vi "Create UI.vi"(8 "error in (no error)":errorcluster, 10 "Instrument.Example in":refnum<class "Instrument.lvclass">, 11 "Instrument.Example UI in":refnum<class "Instrument.PPMS2 UI.lvclass">) -> (0 "error out":errorcluster, 3 "Instrument.Example UI out":refnum<class "Instrument.PPMS2 UI.lvclass">)   [LabVIEW 2016, in "Instrument.PPMS2 UI.lvclass"]
uses:
  Instrument.PPMS2 UI.lvclass
  C:/Program Files (x86)/National Instruments/LabVIEW 2016/vi.lib/JKI/JKI SMO/SMO/SMO.lvclass
  <userlib>/LevyLab/Levylab Instruments/SMOs/Instrument/Instrument.lvclass
  Instrument.PPMS2 UI.lvclass/Instrument.PPMS2 UI.ctl
  <vilib>/JKI/JKI SMO/SMO/SMO.lvclass
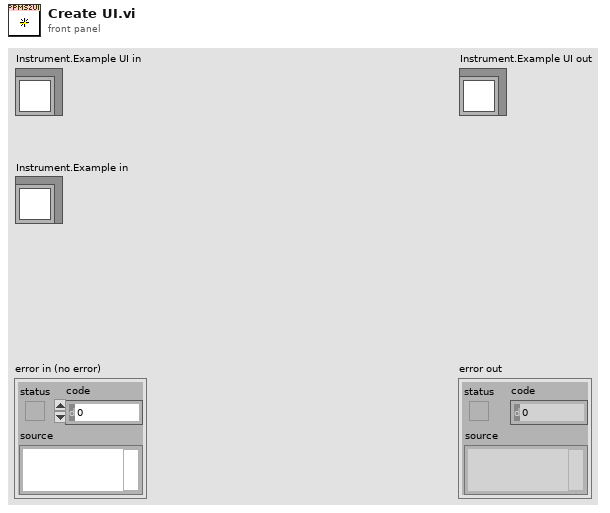
[diagram p1: front panel]
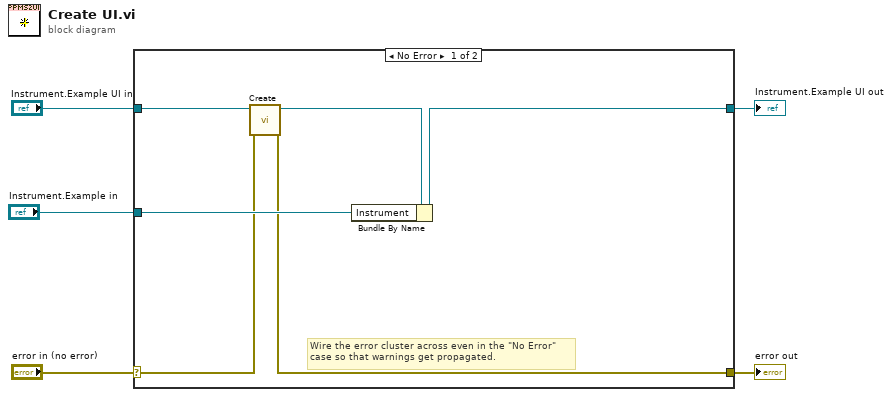
[diagram p0: block diagram]
diagram:
  n1 = case shown="No Error" "error in (no error)" {
    selector: "error in (no error)" -> [w7 w13]
    tunnel: [w6 w13] -> w4
    tunnel: [w11 w12] -> w2
    tunnel: "Instrument.Example UI in" -> [w9 w12]
    tunnel: "Instrument.Example in" -> [w10 _]
    frame No Error {
      # "Wire the error cluster across even in the \"No Error\"\ncase so that warnings get propagated."
      n2 = call <vilib>:"Create.vi"("error in (no error)"=w7, "SMO"=w9) -> ("error out"=w6:errorcluster, "SMO out"=w8:refnum<class "Instrument.PPMS2 UI.lvclass">)  [unwired: 7 in, 1 out]
      n3 = Bundle By Name(cluster=w8, "Instrument"=w10) -> (w11:refnum<class "Instrument.PPMS2 UI.lvclass">)
    }
    frame Error {
    }
  }
  "error out" <- w4
  "Instrument.Example UI out" <- w2
